vi "Set Editor Mode.vi"(8 "Error In":errorcluster, 10 "Mode in":T1, 11 "object in":refnum<class "WebView.JSONEditor.lvclass">) -> (0 "Error Out":errorcluster, 3 "object out":refnum<class "WebView.JSONEditor.lvclass">)   [LabVIEW 2024, in "WebView.JSONEditor.lvclass"]
uses:
  WebView.JSONEditor.lvclass
  C:/Git/WebView-Components/WebView_class/WebView.lvclass
  WebView_class/Editor Mode--enum.ctl
  WebView.JSONEditor.lvclass/WebView.JSONEditor.ctl
  WebView_class/WebView.lvclass
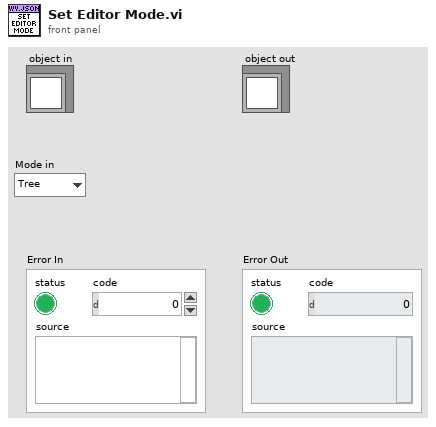
[diagram p1: front panel]
types:
  T1 = typedef "WebView.JSONEditor.lvclass/Editor Mode--enum.ctl" = enum16{"Tree", "View", "Form", "Code", "Text"}
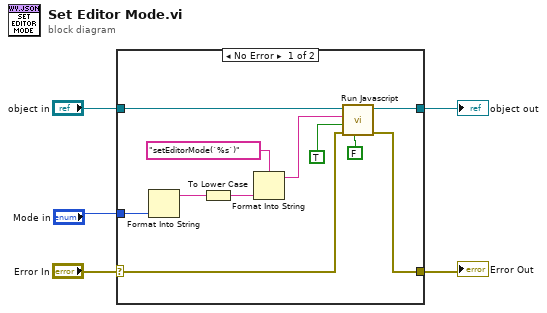
[diagram p0: block diagram]
diagram:
  n1 = case shown="No Error" "Error In" {
    selector: "Error In" -> [w8 w18]
    tunnel: [w7 w18] -> w4
    tunnel: [w11 w17] -> w2
    tunnel: "object in" -> [w12 w17]
    tunnel: "Mode in" -> [w10 _]
    frame No Error {
      n2 = Format Into String(w10) -> (resulting string=w9:string)  [unwired: 3 in, 1 out]
      n3 = To Lower Case(string=w9) -> (all lower case string=w6:string)
      n4 = Format Into String(format string="setEditorMode(`%s`)", w6) -> (resulting string=w14:string)  [unwired: 2 in, 1 out]
      n5 = call "Run Javascript.vi"("Decode Result? (T)"=FALSE, "Error In"=w8, "Fetch Result? (T)"=TRUE, "Javascript in"=w14, "WebView in"=w12) -> ("Error Out"=w7:errorcluster, "WebView out"=w11:refnum<class "WebView.JSONEditor.lvclass">)  [unwired: 4 in, 1 out]
    }
    frame Error {
    }
  }
  "Error Out" <- w4
  "object out" <- w2
